vi "Plant System.vi"(1 "Integrator ?":bool, 2 "output saturation range":cluster{"output high":dbl, "output low":dbl}={"output high"=inf, "output low"=-inf}, 7 "Plant Input":dbl format="%.2f", 11 "dt (s)":dbl=-1.0 format="%.3f", 12 "reinitialize? (F)":bool, 13 "process parameters":T1={"static gain"=2.5, "lag (s)"=2.5, "deadtime (s)"=0.001, "load"=0.0, "deadband"=0.0, "sensor noise"=0.0, "initial PV"=30.0, "plant noise"=0.0} {"plant noise" format="%.2f"; "initial PV" format="%.2f"; "sensor noise" format="%.2f"; "lag (s)" format="%.2f"; "deadtime (s)" format="%.2f"; "deadband" format="%.1f"; "load" format="%.2f"; "static gain" format="%.2f"}) -> (8 "Plant Output":dbl format="%.2f")   [LabVIEW 2023]
doc: "Simulates a physical plant's response; for use with feedback control loops.\n\nAll scale factors are in percent. Lag time is in minutes. Process Deadtime is a true deadtime, measured as a multiple of the loop cycle time. NOTE: this deadtime is dependent upon the interval at which this VI is called. You can modify the algorithm used here to simulate almost any process.\n\nIf more than one plant needs to be simulated simultaneously, save multiple copies of this VI under different names."
uses:
  <vilib>/addons/control/pid/pid.llb/PID Lead-Lag (DBL).vi
  <vilib>/addons/control/pid/NI_PID_pid.lvlib
  <vilib>/addons/control/advanced/NI_AdvCtrl_nonlinear.lvlib
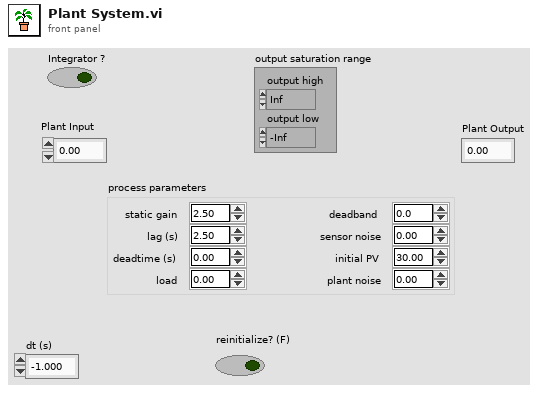
[diagram p1: front panel]
types:
  T1 = cluster{"static gain":dbl, "lag (s)":dbl, "deadtime (s)":dbl, "load":dbl, "deadband":dbl, "sensor noise":dbl, "initial PV":dbl, "plant noise":dbl}
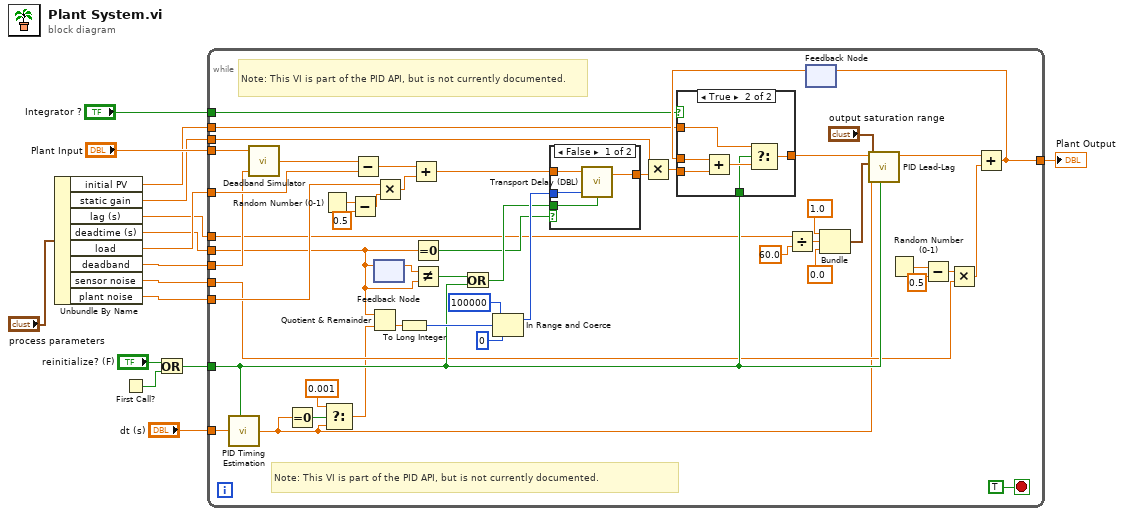
[diagram p0: block diagram]
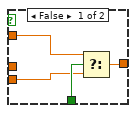
[diagram p3: hidden frame]
diagram:
  n1 = Unbundle By Name("process parameters") -> ("initial PV"=w1:dbl, "static gain"=w5:dbl, "lag (s)"=w3:dbl, "deadtime (s)"=w6:dbl, "load"=w9:dbl, "deadband"=w8:dbl, "sensor noise"=w2:dbl, "plant noise"=w10:dbl)
  n2 = First Call?() -> (First Call?: T/F=w15:bool)
  n3 = Or(x="reinitialize? (F)", y=w15) -> (x .or. y?=w14:bool)
  n4 = while {
    tunnel: w14 -> [w32]
    tunnel: "dt (s)" -> [w33]
    tunnel: [w49] -> w12
    tunnel: w10 -> [w30]
    tunnel: w9 -> [w29]
    tunnel: w8 -> [w28]
    tunnel: "Plant Input" -> [w27]
    tunnel: w6 -> [w20]
    tunnel: w5 -> [w26]
    tunnel: "Integrator ?" -> [w25]
    tunnel: w3 -> [w17]
    tunnel: w2 -> [w24]
    tunnel: w1 -> [w18]
    stop <- TRUE stop-if-true
    # "Note: This VI is part of the PID API, but is not currently documented."
    # "Note: This VI is part of the PID API, but is not currently documented."
    n5 = call <vilib>:"PID Timing Estimation.vi"("Initialize?"=w32, "dt (s) in"=w33) -> ("dt (s) out"=w23:dbl)  [unwired: 7 in]
    n6 = call "Deadband Simulator.vi"("deadband (%)"=w28, "requested pos. (%)"=w27) -> ("actual pos. (%)"=w45:dbl)  [unwired: 1 in]
    n7 = Equal To 0?(x=w23) -> (x = 0?=w35:bool)
    n8 = Random Number (0-1)() -> (number: 0 to 1=w63:dbl)
    n9 = Select(t=0.001, s=w35, f=w23) -> (s? t:f=w21:dbl)
    n10 = Subtract(x=w63, y=0.5) -> (x-y=w31:dbl)
    n11 = Subtract(x=w45, y=w29) -> (x-y=w44:dbl)
    n12 = Quotient & Remainder(x=w20, y=w21) -> (floor(x/y)=w51:dbl)  [unwired: 1 out]
    n13 = feedback-in #1(w20) -> ()
    n14 = feedback #1() -> (w41:dbl)  [unwired: 1 in]
    n15 = Multiply(x=w30, y=w31) -> (x*y=w65:dbl)
    n16 = To Long Integer(number=w51) -> (32bit integer=w39:i32)
    n17 = Add(x=w44, y=w65) -> (x+y=w43:dbl)
    n18 = Equal To 0?(x=w20) -> (x = 0?=w19:bool)
    n19 = Not Equal?(x=w41, y=w20) -> (x != y?=w40:bool)
    n20 = Or(x=w40, y=w32) -> (x .or. y?=w22:bool)
    n21 = In Range and Coerce(upper limit=100000, x=w39, lower limit=0) -> (coerced(x)=w36:i32)  [unwired: 1 out]
    n22 = case shown="False" w19 {
      tunnel: [w69 w70] -> w50
      tunnel: w43 -> [w68 w70]
      tunnel: w36 -> [w67 _]
      tunnel: w22 -> [w66 _]
      frame False {
        n23 = call <vilib>:"Transport Delay (DBL).vi"("initialize"=w66, "delay"=w67, "input point"=w68) -> ("output point"=w69:dbl)  [unwired: 2 in]
      }
      frame True {
      }
    }
    n24 = Multiply(x=w26, y=w50) -> (x*y=w42:dbl)
    n25 = Divide(x=w17, y=60.0) -> (x/y=w47:dbl)
    n26 = feedback #2() -> (w57:dbl)  [unwired: 1 in]
    n27 = case shown="True" w25 {
      tunnel: w42 -> [w73 w80]
      tunnel: [w72 w78] -> w60
      tunnel: w18 -> [w71 w77]
      tunnel: w57 -> [_ w76]
      tunnel: w32 -> [w74 w75]
      frame False {
        n28 = Select(t=w71, s=w74, f=w73) -> (s? t:f=w72:dbl)
      }
      frame True {
        n29 = Add(x=w76, y=w80) -> (x+y=w79:dbl)
        n30 = Select(t=w77, s=w75, f=w79) -> (s? t:f=w78:dbl)
      }
    }
    n31 = Bundle(1.0, w47, 0.0) -> (w58:cluster{dbl, dbl, dbl})  [unwired: 1 in]
    n32 = call-poly <vilib>:"PID Lead-Lag.vi"("reinitialize? (F)"=w32, "dt (s)"=w23, "output range"="output saturation range", "tuning parameters"=w58, "input"=w60) -> ("output"=w53:dbl)  [unwired: 3 in, 1 out]
    n33 = Random Number (0-1)() -> (number: 0 to 1=w56:dbl)
    n34 = Subtract(x=w56, y=0.5) -> (x-y=w55:dbl)
    n35 = Multiply(x=w55, y=w24) -> (x*y=w52:dbl)
    n36 = Add(x=w53, y=w52) -> (x+y=w49:dbl)
    n37 = feedback-in #2(w49) -> ()
  }
  "Plant Output" <- w12
